vi "Begin.vi"(8 "error in":errorcluster) -> (0 "error out":errorcluster)   [LabVIEW 2019]
doc: "Called before other user functions, this VI is expected to open initial I/O refnums, load in file data, and do all program initialization. Notice that the <B>error out</B> terminal is simply used for data flow. Wiring it to other structures or subVIs ensures that this VI runs first."
uses:
  <vilib>/Rock Robotics/WPI/DriverStation/WPI_DriverStationRobotMode2.ctl
  <vilib>/Rock Robotics/WPI/Joystick/WPI_JoystickDeviceEnum.ctl
  <vilib>/Rock Robotics/WPI/ThirdParty/Phoenix-LabVIEW/Motor Controller/Controls/CTRE_Phoenix_MotorControl_NeutralMode.ctl
  <vilib>/Rock Robotics/WPI/ThirdParty/Phoenix-LabVIEW/Motor Controller/Controls/CTRE_Phoenix_MotorControl_FeedbackDevice.ctl
  <vilib>/Rock Robotics/WPI/SafetyOutput/WPI_SafetyOutputConfigMenu.ctl
  Robot Global Data.vi
  <vilib>/Rock Robotics/Network Tables/NT Write String Array.vi
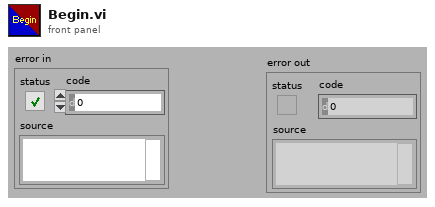
[diagram p1: front panel]
types:
  T1 = typedef "WPI_SafetyOutputConfigMenu.ctl" = enum16{"Enable", "Disable"}
  T2 = typedef "CTRE_Phoenix_MotorControl_FeedbackDevice.ctl" = i8
  T3 = typedef "CTRE_Phoenix_MotorControl_NeutralMode.ctl" = enum8{"EEPROMSetting", "Override to Coast", "Override to Brake"}
  T4 = enum16{"FollowerType_PercentOutput", "FollowerType_AuxOutput1"}
  T5 = typedef "WPI_JoystickDeviceEnum.ctl" = enum16{"USB 0", "USB 1", "USB 2", "USB 3", "USB 4", "USB 5"}
  T6 = typedef "WPI_DriverStationRobotMode2.ctl" = enum16{"Autonomous Disabled", "Autonomous Enabled", "Teleop Disabled", "Teleop Enabled", "Disconnected", "Finish", "Test Disabled", "Test Enabled", "Emergency Stopped"}
  T7 = typedef "WPI_JoystickDevRef.ctl" = cluster{"Device":T5}
  T8 = typedef "WPI_MotorControlDeviceRef.ctl" = cluster{"DeviceStatus":errorcluster, "Type":T9, "PWM":cluster{"PWM Channel":T10, "DeadBand":T11}, "CAN":cluster{"Device Number":u8, "SetOutput VI Ref":variant, "GetOutput VI Ref":variant, "Enable VI Ref":variant, "Disable VI Ref":variant, "Data":variant}, "Invert":bool, "DIO PWM":cluster{"PWM \"Enable\" Channel":T10, "DIOChannel":T12, "PWM Rate":dbl}}
  T9 = typedef "WPI_MotorControlType.ctl" = enum16{"PWM", "CAN", "DIO PWM"}
  T10 = typedef "FPGA_DIOPWMChannel.ctl" = enum8{"PWM 0", "PWM 1", "PWM 2", "PWM 3", "PWM 4", "PWM 5", "PWM 6", "PWM 7", "PWM 8", "PWM 9", "PWM MXP 0", "PWM MXP 1", "PWM MXP 2", "PWM MXP 3", "PWM MXP 4", "PWM MXP 5", "PWM MXP 6", "PWM MXP 7", "PWM MXP 8", "PWM MXP 9", "Invalid"}
  T11 = typedef "WPI_PWMDeadband.ctl" = cluster{"Name":string, "maxPositivePwm":i32, "minPositivePwm":i32, "centerPwm":i32, "maxNegativePwm":i32, "minNegativePwm":i32, "angularRange":u16}
  T12 = typedef "FPGA_DIOChannel.ctl" = enum8{"DIO 0", "DIO 1", "DIO 2", "DIO 3", "DIO 4", "DIO 5", "DIO 6", "DIO 7", "DIO 8", "DIO 9", "DIO MXP 0", "DIO MXP 1", "DIO MXP 2", "DIO MXP 3", "DIO MXP 4", "DIO MXP 5", "DIO MXP 6", "DIO MXP 7", "DIO MXP 8", "DIO MXP 9", "DIO MXP 10", "DIO MXP 11", "DIO MXP 12", "DIO MXP 13", "DIO MXP 14", "DIO MXP 15", "SPI Port CS1", "SPI Port CS2", "SPI Port CS3", "SPI Port MISO", "SPI Port MOSI", "Invalid"}
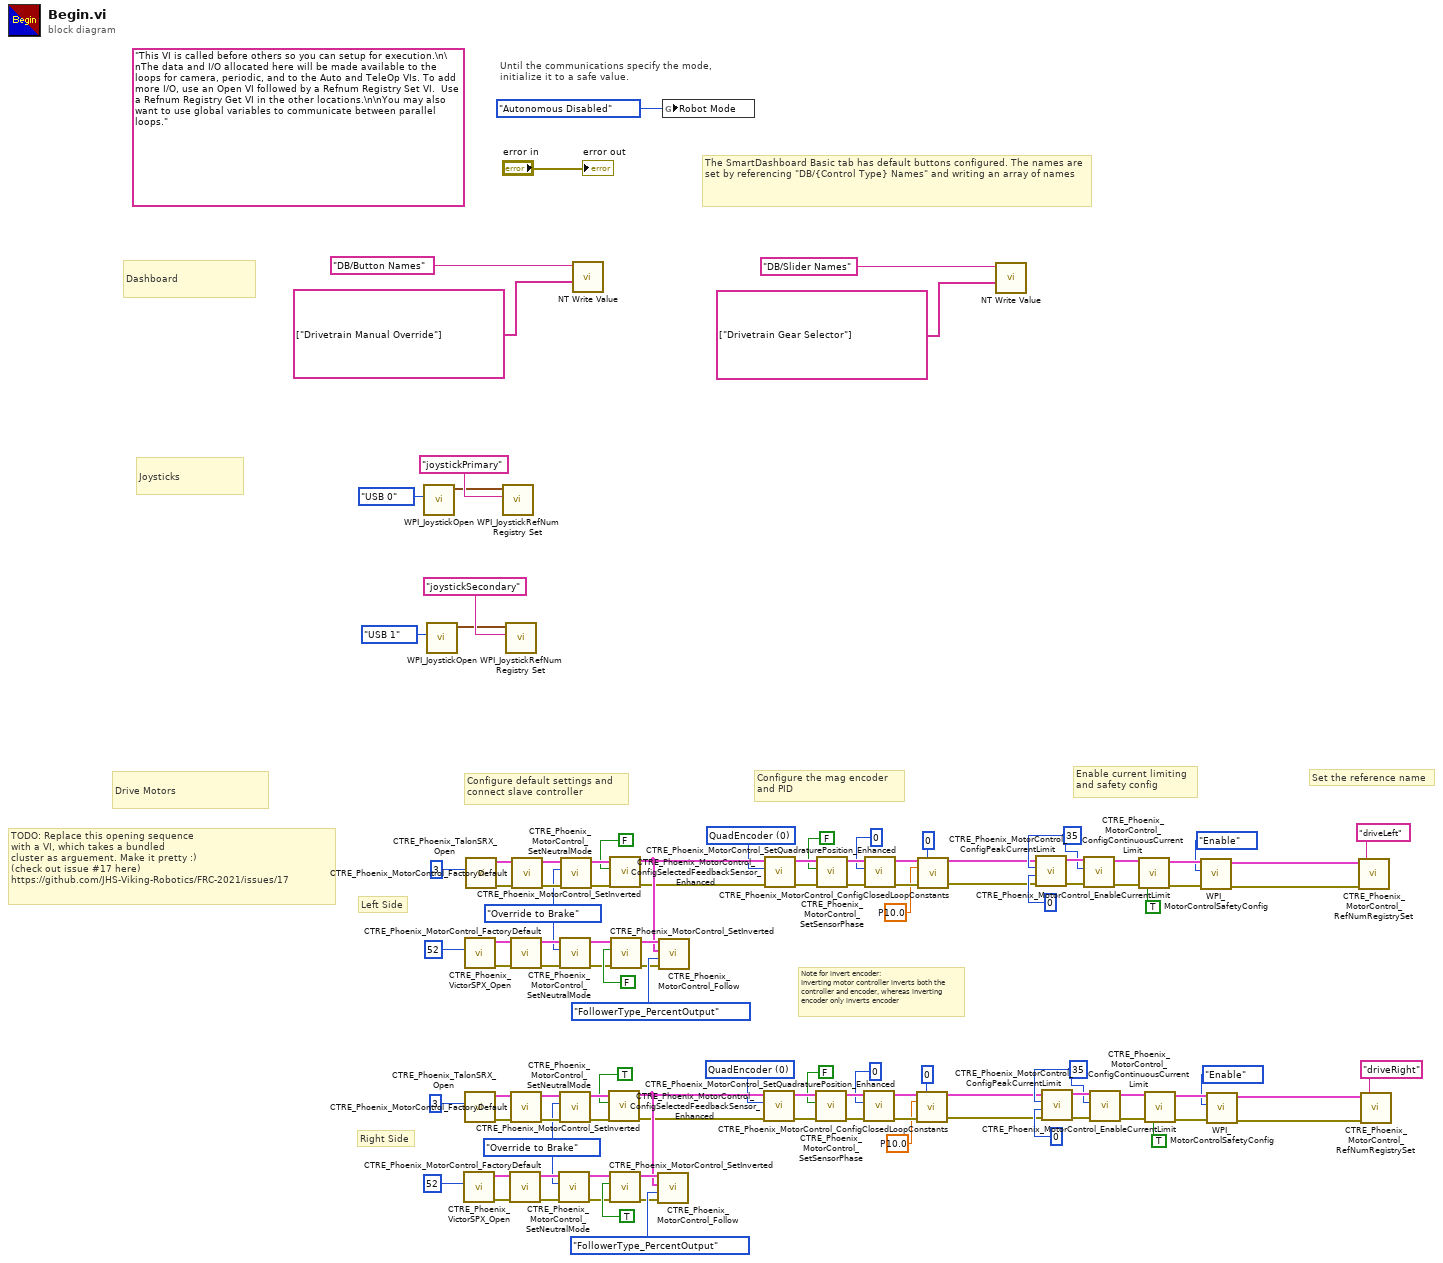
[diagram p0: block diagram]
diagram:
  w17 = 35 ("Peak Current (Amps)")
  w29 = 35 ("Peak Current (Amps)")
  w35 = 10.0  # P
  w45 = T2 0 items=["QuadEncoder"=0, "Analog"=2, "Tachometer"=4, "Pulse Width Encoded Position"=8, "Sensor Sum (S0 + S1)"=9, "Sensor Difference (D0 - D1)"=10, "Remote Source 0"=11, "Remote Source 1"=12, "Software Emulated"=15] ("Feedback Device")
  w47 = CTRE_Phoenix_MotorControl_NeutralMode."Override to Brake" ("Motor Control Neutral Mode")
  w69 = 10.0  # P
  w79 = T2 0 items=["QuadEncoder"=0, "Analog"=2, "Tachometer"=4, "Pulse Width Encoded Position"=8, "Sensor Sum (S0 + S1)"=9, "Sensor Difference (D0 - D1)"=10, "Remote Source 0"=11, "Remote Source 1"=12, "Software Emulated"=15] ("Feedback Device")
  w81 = CTRE_Phoenix_MotorControl_NeutralMode."Override to Brake" ("Motor Control Neutral Mode")
  (unwired) "This VI is called before others so you can setup for execution.\n\nThe data and I/O allocated here will be made available to the loops for camera, periodic, and to the Auto and TeleOp VIs. To add more I/O, use an Open VI followed by a Refnum Registry Set VI.  Use a Refnum Registry Get VI in the other locations.\n\nYou may also want to use global variables to communicate between parallel loops."
  # "The SmartDashboard Basic tab has default buttons configured. The names are set by referencing \"DB/{Control Type} Names\" and writing an array of names"
  # "Dashboard"
  # "Enable current limiting\nand safety config"
  # "Note for invert encoder:\nInverting motor controller inverts both the\ncontroller and encoder, whereas inverting\nencoder only inverts encoder"
  # "Right Side"
  # "Set the reference name"
  # "Left Side"
  # "Drive Motors"
  # "TODO: Replace this opening sequence\nwith a VI, which takes a bundled\ncluster as arguement. Make it pretty :)\n(check out issue #17 here)\nhttps://github.com/JHS-Viking-Robotics/FRC-2021/issues/17"
  # "Configure the mag encoder\nand PID"
  # "Configure default settings and\nconnect slave controller"
  # "Joysticks"
  # "Until the communications specify the mode,\ninitialize it to a safe value."
  n1 = call <vilib>:"WPI_JoystickOpen.vi"("JoystickDevice"=WPI_JoystickDeviceEnum."USB 0") -> ("JoystickDevRef"=w106:T7)  [unwired: 10 in]
  n2 = call <vilib>:"WPI_JoystickOpen.vi"("JoystickDevice"=WPI_JoystickDeviceEnum."USB 1") -> ("JoystickDevRef"=w102:T7)  [unwired: 10 in]
  n3 = call <vilib>:"CTRE_Phoenix_VictorSPX_Open.vi"("Device Number"=u8 52) -> ("error out"=w61:errorcluster, "CAN Talon SRX Ref"=w62:T8)  [unwired: 9 in]
  n4 = call <vilib>:"CTRE_Phoenix_VictorSPX_Open.vi"("Device Number"=u8 52) -> ("error out"=w95:errorcluster, "CAN Talon SRX Ref"=w96:T8)  [unwired: 9 in]
  n5 = call <vilib>:"CTRE_Phoenix_TalonSRX_Open.vi"("Device Number"=u8 3) -> ("error out"=w64:errorcluster, "CAN Talon SRX Ref"=w65:T8)  [unwired: 9 in]
  n6 = call <vilib>:"CTRE_Phoenix_TalonSRX_Open.vi"("Device Number"=u8 3) -> ("error out"=w98:errorcluster, "CAN Talon SRX Ref"=w99:T8)  [unwired: 9 in]
  n7 = call <vilib>:"WPI_JoystickRefNum Registry Set.vi"("refnum name"="joystickPrimary", "JoystickDevRef"=w106) -> ()  [unwired: 8 in, 2 out]
  n8 = call <vilib>:"WPI_JoystickRefNum Registry Set.vi"("refnum name"="joystickSecondary", "JoystickDevRef"=w102) -> ()  [unwired: 8 in, 2 out]
  n9 = call <vilib>:"CTRE_Phoenix_MotorControl_FactoryDefault.vi"("error in"=w61, "PhoenixMotorControlDevRef"=w62) -> ("error out"=w51:errorcluster, "PhoenixMotorControlDevRef"=w49:T8)  [unwired: 8 in]
  n10 = call <vilib>:"CTRE_Phoenix_MotorControl_FactoryDefault.vi"("error in"=w95, "PhoenixMotorControlDevRef"=w96) -> ("error out"=w85:errorcluster, "PhoenixMotorControlDevRef"=w83:T8)  [unwired: 8 in]
  n11 = call <vilib>:"CTRE_Phoenix_MotorControl_FactoryDefault.vi"("error in"=w64, "PhoenixMotorControlDevRef"=w65) -> ("error out"=w59:errorcluster, "PhoenixMotorControlDevRef"=w58:T8)  [unwired: 8 in]
  n12 = call <vilib>:"CTRE_Phoenix_MotorControl_FactoryDefault.vi"("error in"=w98, "PhoenixMotorControlDevRef"=w99) -> ("error out"=w93:errorcluster, "PhoenixMotorControlDevRef"=w92:T8)  [unwired: 8 in]
  n13 = call <vilib>:"CTRE_Phoenix_MotorControl_SetNeutralMode.vi"("error in (no error)"=w51, "Motor Control Neutral Mode"=w47, "PhoenixMotorControlDevRef"=w49) -> ("error out"=w50:errorcluster, "PhoenixMotorControlDevRef"=w48:T8)  [unwired: 7 in]
  n14 = call <vilib>:"CTRE_Phoenix_MotorControl_SetNeutralMode.vi"("error in (no error)"=w85, "Motor Control Neutral Mode"=w81, "PhoenixMotorControlDevRef"=w83) -> ("error out"=w84:errorcluster, "PhoenixMotorControlDevRef"=w82:T8)  [unwired: 7 in]
  n15 = call <vilib>:"CTRE_Phoenix_MotorControl_SetNeutralMode.vi"("error in (no error)"=w59, "Motor Control Neutral Mode"=w47, "PhoenixMotorControlDevRef"=w58) -> ("error out"=w57:errorcluster, "PhoenixMotorControlDevRef"=w56:T8)  [unwired: 7 in]
  n16 = call <vilib>:"CTRE_Phoenix_MotorControl_SetNeutralMode.vi"("error in (no error)"=w93, "Motor Control Neutral Mode"=w81, "PhoenixMotorControlDevRef"=w92) -> ("error out"=w91:errorcluster, "PhoenixMotorControlDevRef"=w90:T8)  [unwired: 7 in]
  n17 = call-poly <vilib>:"NT Write Value.vi"("String Array"=string[] ["Drivetrain Manual Override"], "Name"="DB/Button Names") -> ()  [unwired: 9 in, 1 out]
  n18 = call <vilib>:"CTRE_Phoenix_MotorControl_SetInverted.vi"("error in (no error)"=w57, "Invert?"=TRUE, "PhoenixMotorControlDevRef"=w56) -> ("error out"=w44:errorcluster, "PhoenixMotorControlDevRef"=w46:T8)  [unwired: 7 in]
  n19 = call <vilib>:"CTRE_Phoenix_MotorControl_SetInverted.vi"("error in (no error)"=w91, "Invert?"=FALSE, "PhoenixMotorControlDevRef"=w90) -> ("error out"=w78:errorcluster, "PhoenixMotorControlDevRef"=w80:T8)  [unwired: 7 in]
  n20 = call <vilib>:"CTRE_Phoenix_MotorControl_SetInverted.vi"("error in (no error)"=w50, "Invert?"=TRUE, "PhoenixMotorControlDevRef"=w48) -> ("error out"=w53:errorcluster, "PhoenixMotorControlDevRef"=w52:T8)  [unwired: 7 in]
  n21 = call <vilib>:"CTRE_Phoenix_MotorControl_SetInverted.vi"("error in (no error)"=w84, "Invert?"=FALSE, "PhoenixMotorControlDevRef"=w82) -> ("error out"=w87:errorcluster, "PhoenixMotorControlDevRef"=w86:T8)  [unwired: 7 in]
  n22 = call <vilib>:"CTRE_Phoenix_MotorControl_Follow.vi"("error in (no error)"=w53, "FollowerType"=T4."FollowerType_PercentOutput", "Master Controller to Follow"=w46, "PhoenixMotorControlDevRef"=w52) -> ()  [unwired: 6 in, 2 out]
  n23 = call <vilib>:"CTRE_Phoenix_MotorControl_Follow.vi"("error in (no error)"=w87, "FollowerType"=T4."FollowerType_PercentOutput", "Master Controller to Follow"=w80, "PhoenixMotorControlDevRef"=w86) -> ()  [unwired: 6 in, 2 out]
  n24 = global write "Robot Global Data.vi" "Robot Mode"(WPI_DriverStationRobotMode2."Autonomous Disabled" ("Robot Mode")) -> ()
  n25 = call <vilib>:"CTRE_Phoenix_MotorControl_ConfigSelectedFeedbackSensor_Enhanced.vi"("error in (no error)"=w44, "Feedback Device"=w45, "PhoenixMotorControlDevRef"=w46) -> ("error out"=w43:errorcluster, "PhoenixMotorControlDevRef"=w42:T8)  [unwired: 7 in]
  n26 = call <vilib>:"CTRE_Phoenix_MotorControl_ConfigSelectedFeedbackSensor_Enhanced.vi"("error in (no error)"=w78, "Feedback Device"=w79, "PhoenixMotorControlDevRef"=w80) -> ("error out"=w77:errorcluster, "PhoenixMotorControlDevRef"=w76:T8)  [unwired: 7 in]
  n27 = call <vilib>:"CTRE_Phoenix_MotorControl_SetSensorPhase.vi"("error in (no error)"=w43, "PhaseSensor"=FALSE, "PhoenixMotorControlDevRef"=w42) -> ("error out"=w40:errorcluster, "PhoenixMotorControlDevRef"=w39:T8)  [unwired: 7 in]
  n28 = call <vilib>:"CTRE_Phoenix_MotorControl_SetSensorPhase.vi"("error in (no error)"=w77, "PhaseSensor"=FALSE, "PhoenixMotorControlDevRef"=w76) -> ("error out"=w74:errorcluster, "PhoenixMotorControlDevRef"=w73:T8)  [unwired: 7 in]
  n29 = call <vilib>:"CTRE_Phoenix_MotorControl_SetQuadraturePosition_Enhanced.vi"("error in (no error)"=w40, "New Position"=0, "PhoenixMotorControlDevRef"=w39) -> ("error out"=w36:errorcluster, "PhoenixMotorControlDevRef"=w37:T8)  [unwired: 7 in]
  n30 = call <vilib>:"CTRE_Phoenix_MotorControl_SetQuadraturePosition_Enhanced.vi"("error in (no error)"=w74, "New Position"=0, "PhoenixMotorControlDevRef"=w73) -> ("error out"=w70:errorcluster, "PhoenixMotorControlDevRef"=w71:T8)  [unwired: 7 in]
  n31 = call <vilib>:"CTRE_Phoenix_MotorControl_ConfigClosedLoopConstants.vi"("PhoenixMotorControlDevRef"=w37, "slotIdx"=0, "P"=w35, "error in (no error)"=w36) -> ("PhoenixMotorControlDevRef"=w22:T8, "error out"=w21:errorcluster)  [unwired: 10 in]
  n32 = call <vilib>:"CTRE_Phoenix_MotorControl_ConfigClosedLoopConstants.vi"("PhoenixMotorControlDevRef"=w71, "slotIdx"=0, "P"=w69, "error in (no error)"=w70) -> ("PhoenixMotorControlDevRef"=w10:T8, "error out"=w9:errorcluster)  [unwired: 10 in]
  n33 = call-poly <vilib>:"NT Write Value.vi"("String Array"=string[] ["Drivetrain Gear Selector"], "Name"="DB/Slider Names") -> ()  [unwired: 9 in, 1 out]
  n34 = call <vilib>:"CTRE_Phoenix_MotorControl_ConfigPeakCurrentLimit.vi"("error in (no error)"=w9, "Peak Current Maximum Duration (ms)"=0, "Peak Current (Amps)"=w17, "PhoenixMotorControlDevRef"=w10) -> ("error out"=w18:errorcluster, "PhoenixMotorControlDevRef"=w19:T8)  [unwired: 6 in]
  n35 = call <vilib>:"CTRE_Phoenix_MotorControl_ConfigPeakCurrentLimit.vi"("error in (no error)"=w21, "Peak Current Maximum Duration (ms)"=0, "Peak Current (Amps)"=w29, "PhoenixMotorControlDevRef"=w22) -> ("error out"=w30:errorcluster, "PhoenixMotorControlDevRef"=w31:T8)  [unwired: 6 in]
  n36 = call <vilib>:"CTRE_Phoenix_MotorControl_ConfigContinuousCurrentLimit.vi"("error in (no error)"=w18, "Continuous Current Limit (Amps)"=w17, "PhoenixMotorControlDevRef"=w19) -> ("error out"=w15:errorcluster, "PhoenixMotorControlDevRef"=w16:T8)  [unwired: 7 in]
  n37 = call <vilib>:"CTRE_Phoenix_MotorControl_ConfigContinuousCurrentLimit.vi"("error in (no error)"=w30, "Continuous Current Limit (Amps)"=w29, "PhoenixMotorControlDevRef"=w31) -> ("error out"=w27:errorcluster, "PhoenixMotorControlDevRef"=w28:T8)  [unwired: 7 in]
  n38 = call <vilib>:"CTRE_Phoenix_MotorControl_EnableCurrentLimit.vi"("error in (no error)"=w15, "Enable Current Limit?"=TRUE, "PhoenixMotorControlDevRef"=w16) -> ("error out"=w12:errorcluster, "PhoenixMotorControlDevRef"=w13:T8)  [unwired: 7 in]
  n39 = call <vilib>:"CTRE_Phoenix_MotorControl_EnableCurrentLimit.vi"("error in (no error)"=w27, "Enable Current Limit?"=TRUE, "PhoenixMotorControlDevRef"=w28) -> ("error out"=w24:errorcluster, "PhoenixMotorControlDevRef"=w25:T8)  [unwired: 7 in]
  n40 = call <vilib>:"WPI_MotorControlSafetyConfig.vi"("error in (no error)"=w12, "mode"=WPI_SafetyOutputConfigMenu."Enable", "MotorControlDevRef"=w13) -> ("error out"=w7:errorcluster, "MotorControlDevRef"=w8:T8)  [unwired: 7 in]
  n41 = call <vilib>:"WPI_MotorControlSafetyConfig.vi"("error in (no error)"=w24, "mode"=WPI_SafetyOutputConfigMenu."Enable", "MotorControlDevRef"=w25) -> ("error out"=w5:errorcluster, "MotorControlDevRef"=w6:T8)  [unwired: 7 in]
  n42 = call <vilib>:"CTRE_Phoenix_MotorControl_RefNumRegistrySet.vi"("error in (no error)"=w7, "refnum name"="driveLeft", "PhoenixMotorControlDevRef"=w8) -> ()  [unwired: 7 in, 2 out]
  n43 = call <vilib>:"CTRE_Phoenix_MotorControl_RefNumRegistrySet.vi"("error in (no error)"=w5, "refnum name"="driveRight", "PhoenixMotorControlDevRef"=w6) -> ()  [unwired: 7 in, 2 out]
  "error out" <- "error in"
